vi "FRCts20_Backend_Test_SNS_Publish.vi"(8 "error in (no error)":errorcluster) -> (0 "error out":errorcluster, 1 "Time (ms)":u32, 2 "Status":string, 3 "Event Out":T1, 5 "Success":bool)   [LabVIEW 2014, in "FRCts20_Backend_TestCode.lvlib"]
uses:
  FRCts20_Backend_TestCode.lvlib
  FRCts20_Backend_API/FRCts20_Backend_API_SNS.ctl
  FRCts20_Backend_API/FRCts20_Backend_API_Command_SNS.ctl
  FRCts20_Backend_API/FRCts20_Backend_API_SNS.vi
  FRCts20_Backend_API/FRCts20_Backend_API.lvlib
panel:
  in  "Main Message":string
  in  "Event Name":string
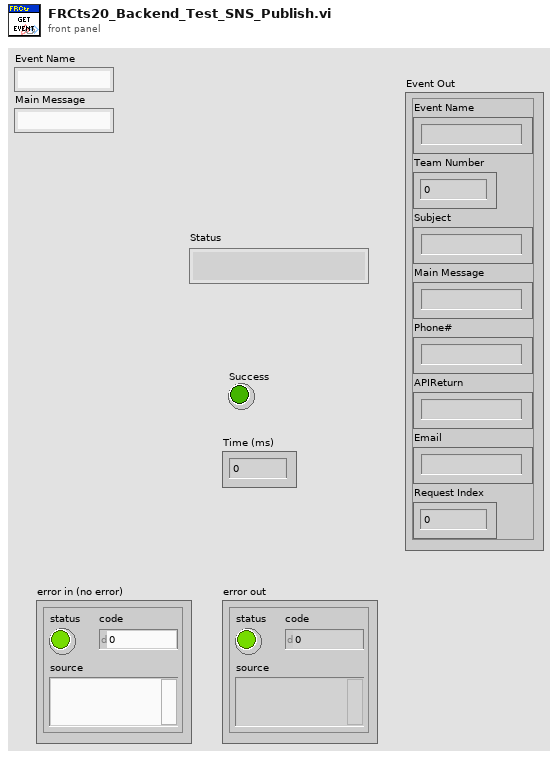
[diagram p1: front panel]
types:
  T1 = typedef "FRCts20_Backend_API.lvlib/FRCts20_Backend_API_SNS.ctl" = cluster{"Event Name":string, "Team Number":u32, "Subject":string, "Main Message":string, "Phone#":string, "APIReturn":string, "Email":string, "Request Index":u32}
  T2 = typedef "FRCts20_Backend_API.lvlib/FRCts20_Backend_API_Command_SNS.ctl" = string
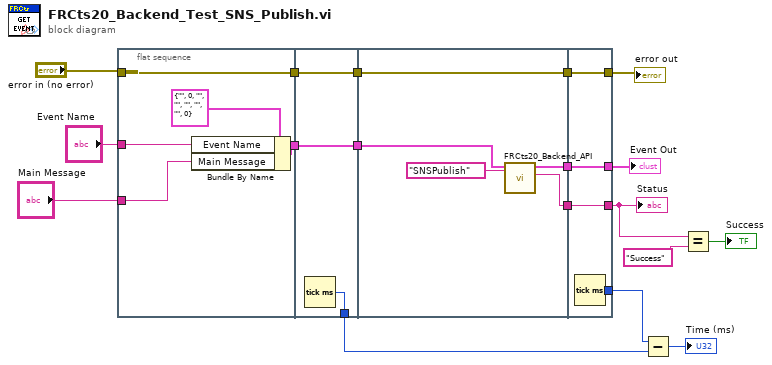
[diagram p0: block diagram]
diagram:
  n1 = flat-sequence {
    tunnel: "error in (no error)" -> [w23]
    tunnel: [w23] -> w16
    tunnel: [w21] -> w4
    tunnel: "Event Name" -> [w20]
    tunnel: "Main Message" -> [w19]
    tunnel: [w26] -> w9
    tunnel: [w25] -> w15
    tunnel: w16 -> [w25]
    tunnel: [w24] -> w5
    tunnel: w4 -> [w24]
    tunnel: [w31] -> w14
    tunnel: w15 -> [w31]
    tunnel: [w30] -> w8
    tunnel: [w29] -> w7
    tunnel: w5 -> [w27]
    tunnel: [w35] -> w10
    tunnel: [w34] -> w12
    tunnel: w14 -> [w34]
    tunnel: [w33] -> w2
    tunnel: w8 -> [w33]
    tunnel: [w32] -> w6
    tunnel: w7 -> [w32]
    frame #0 {
      n2 = Bundle By Name(cluster=T1 {"Event Name"="", "Team Number"=0, "Subject"="", "Main Message"="", "Phone#"="", "APIReturn"="", "Email"="", "Request Index"=0} ("Event In"), "Event Name"=w20, "Main Message"=w19) -> (w21:T1)
    }
    frame #1 {
      n3 = Tick Count (ms)() -> (millisecond timer value=w26:u32)
    }
    frame #2 {
      n4 = call-poly "FRCts20_Backend_API.vi"("SNS"=T2 "SNSPublish", "Event In"=w27) -> ("Status"=w29:string, "Event Out"=w30:T1)  [unwired: 7 in, 1 out]
    }
    frame #3 {
      n5 = Tick Count (ms)() -> (millisecond timer value=w35:u32)
    }
  }
  n6 = Subtract(x=w10, y=w9) -> (x-y=→"Time (ms)":u32)
  n7 = Equal?(x=w6, y="Success") -> (x = y?=→"Success":bool)
  "Event Out" <- w2
  "Status" <- w6
  "error out" <- w12
